vi "Init.vi"(8 "error in (no error)":errorcluster) -> (0 "error out":errorcluster, 3 "VectoService out":refnum<class "VectoInfo.lvclass">)   [LabVIEW 2020, in "Vecto.lvlib" / "VectoInfo.lvclass"]
uses:
  VectoInfo.lvclass
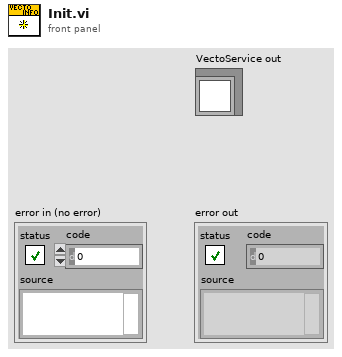
[diagram p1: front panel]
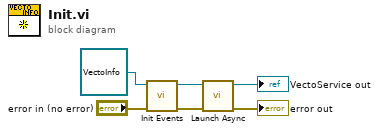
[diagram p0: block diagram]
diagram:
  n1 = call "Init Events.vi"("error in (no error)"="error in (no error)", "VectoService in"=refnum<class "VectoInfo.lvclass"> refnum) -> ("error out"=w4:errorcluster, "VectoService out"=w2:refnum<class "VectoInfo.lvclass">)  [unwired: 8 in]
  n2 = call "Launch Async.vi"("error in (no error)"=w4, "VectoService in"=w2) -> ("error out"=→"error out":errorcluster, "VectoService out"=→"VectoService out":refnum<class "VectoInfo.lvclass">)  [unwired: 8 in]
